vi "Actor Core.vi"(8 "error in":errorcluster, 11 "Main Dock View in":refnum<class "Main Dock View.lvclass">) -> (0 "error out":errorcluster, 3 "Actor out":refnum<class "Actor.lvclass">)   [LabVIEW 2020, in "Main Dock View.lvlib" / "Main Dock View.lvclass"]
doc: "(<B>Filename</B>: Actor Framework.lvlib:Actor.lvclass:Actor Core.vi)\n\nReceives messages to the actor, reacts to them, and initiates any error handling that may shut the actor down.\n\nDescendant classes may override this VI to append parallel tasks for the actor to complete while it handles messages. Overrides use the Call Parent Method node."
uses:
  Main Dock View.lvclass
  C:/Program Files/National Instruments/LabVIEW 2020/vi.lib/ActorFramework/Actor/Actor.lvclass
  <vilib>/ActorFramework/Actor/Actor.lvclass
  <vilib>/ActorFramework/Actor/Actor.lvclass/Actor.ctl
  <vilib>/ActorFrameworkMVC/View Controller/View Controller Messages/Set Splitter Msg/Set Splitter Msg.lvclass/Set Splitter Msg.ctl
  <vilib>/ActorFramework/Message Enqueuer/Message Enqueuer.lvclass/Message Enqueuer.ctl
  <vilib>/ActorFrameworkMVC/View Controller/View Controller Messages/Move Splitter Msg/Move Splitter Msg.lvclass/Move Splitter Msg.ctl
  <vilib>/ActorFrameworkMVC/View Controller/View Controller Messages/Set Subpanel Msg/Set Subpanel Msg.lvclass/Set Subpanel Msg.ctl
  <vilib>/ActorFramework/Message Enqueuer/Enqueue.vi
  <vilib>/ActorFrameworkMVC/View Controller/View Controller Messages/Set Splitter Msg/Set Splitter Msg.lvclass
  C:/Program Files/National Instruments/LabVIEW 2020/vi.lib/ActorFramework/Message/Message.lvclass
  <vilib>/ActorFrameworkMVC/View Controller/View Controller Messages/Move Splitter Msg/Move Splitter Msg.lvclass
  <vilib>/ActorFrameworkMVC/View Controller/View Controller Messages/Set Subpanel Msg/Set Subpanel Msg.lvclass
  <vilib>/ActorFramework/Message Priority Queue/Priority Enqueue.vi
  <vilib>/ActorFrameworkMVC/Abstract View/Abstract View/Abstract View.lvclass
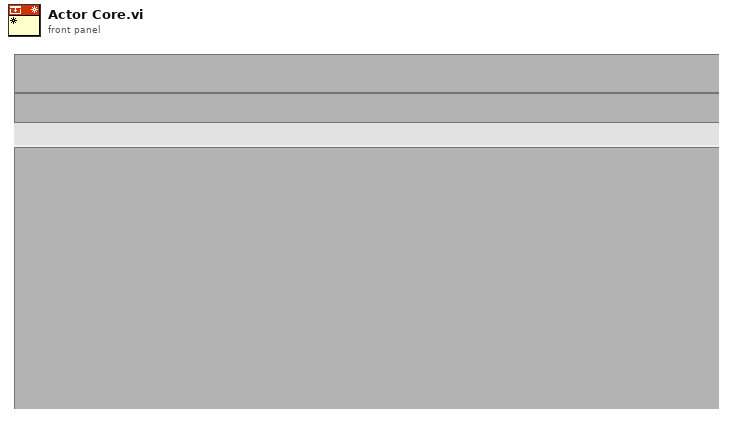
[diagram p1: front panel]
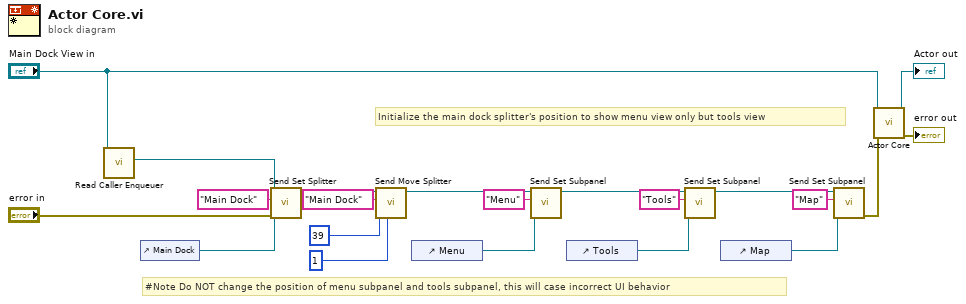
[diagram p0: block diagram]
diagram:
  # "#Note Do NOT change the position of menu subpanel and tools subpanel, this will case incorrect UI behavior"
  # "Initialize the main dock splitter's position to show menu view only but tools view"
  n1 = call <vilib>:"Read Caller Enqueuer.vi"("Actor"="Main Dock View in") -> ("Caller Enqueuer"=w19:refnum<class "Message Enqueuer.lvclass">)  [unwired: 10 in]
  n2 = control-ref of="Main Dock"() -> (w14:refnum<vi>)
  n3 = call <vilib>:"Send Set Splitter.vi"("error in (no error)"="error in", "Splitter Reference"=w14, "Splitter Name"="Main Dock", "Message Enqueuer"=w19) -> ("Message Enqueuer out"=w20:refnum<class "Message Enqueuer.lvclass">)  [unwired: 6 in, 1 out]
  n4 = call <vilib>:"Send Move Splitter.vi"("Loop Number (16)"=1, "Splitter Position"=39, "Splitter Name"="Main Dock", "Message Enqueuer"=w20) -> ("Message Enqueuer out"=w12:refnum<class "Message Enqueuer.lvclass">)  [unwired: 6 in, 1 out]
  n5 = control-ref of="Menu"() -> (w2:refnum<vi>)
  n6 = call <vilib>:"Send Set Subpanel.vi"("SubPanel Reference"=w2, "Subpanel Name"="Menu", "Message Enqueuer"=w12) -> ("Message Enqueuer out"=w7:refnum<class "Message Enqueuer.lvclass">)  [unwired: 7 in, 1 out]
  n7 = control-ref of="Tools"() -> (w1:refnum<vi>)
  n8 = call <vilib>:"Send Set Subpanel.vi"("SubPanel Reference"=w1, "Subpanel Name"="Tools", "Message Enqueuer"=w7) -> ("Message Enqueuer out"=w6:refnum<class "Message Enqueuer.lvclass">)  [unwired: 7 in, 1 out]
  n9 = control-ref of="Map"() -> (w13:refnum<vi>)
  n10 = call <vilib>:"Send Set Subpanel.vi"("SubPanel Reference"=w13, "Subpanel Name"="Map", "Message Enqueuer"=w6) -> ("error out"=w3:errorcluster)  [unwired: 7 in, 1 out]
  n11 = call-parent "Actor Core.vi"("error in"=w3, "Abstract View in"="Main Dock View in") -> ("error out"=→"error out":errorcluster, "Actor out"=→"Actor out":refnum<class "Actor.lvclass">)  [unwired: 8 in]
